vi "SUB-BLE Rx data (Debug)-CDC_KH2.vi"(8 "data in":u8[](array[numeric]) format="%2x") -> (2 "CDC debug":T1 caption="CDC Debugging data" {"Right Wing-C, C6/C0" format="%#.9f"; "Right Wing-B, C5/C0" format="%#.9f"; "Right Wing-A, C4/C0" format="%#.9f"; "Left Wing-C, C3/C0" format="%#.9f"; "Left Wing-B, C2/C0" format="%#.9f"; "Left Wing-A, C1/C0" format="%#.9f"}, 3 "CDC mon":T1 caption="CDC Monitoring data" {"Right Wing-C, C6/C0" format="%#.9f"; "Right Wing-B, C5/C0" format="%#.9f"; "Right Wing-A, C4/C0" format="%#.9f"; "Left Wing-C, C3/C0" format="%#.9f"; "Left Wing-B, C2/C0" format="%#.9f"; "Left Wing-A, C1/C0" format="%#.9f"})   [LabVIEW 2015]
doc: "Use this template to create an application that executes repeatedly until you click the Stop button. This template polls the state of the Stop button and does not use events. Use the Top-Level Application template (not available in the Base package) to create a single-loop application with event handling."
panel:
  out "BLE Packet (buf)":u8[](array[numeric])
  out "BLE Packet (data)":u8[](array[numeric])
  # "BLE 수신 데이터를 처리: Debugging data"
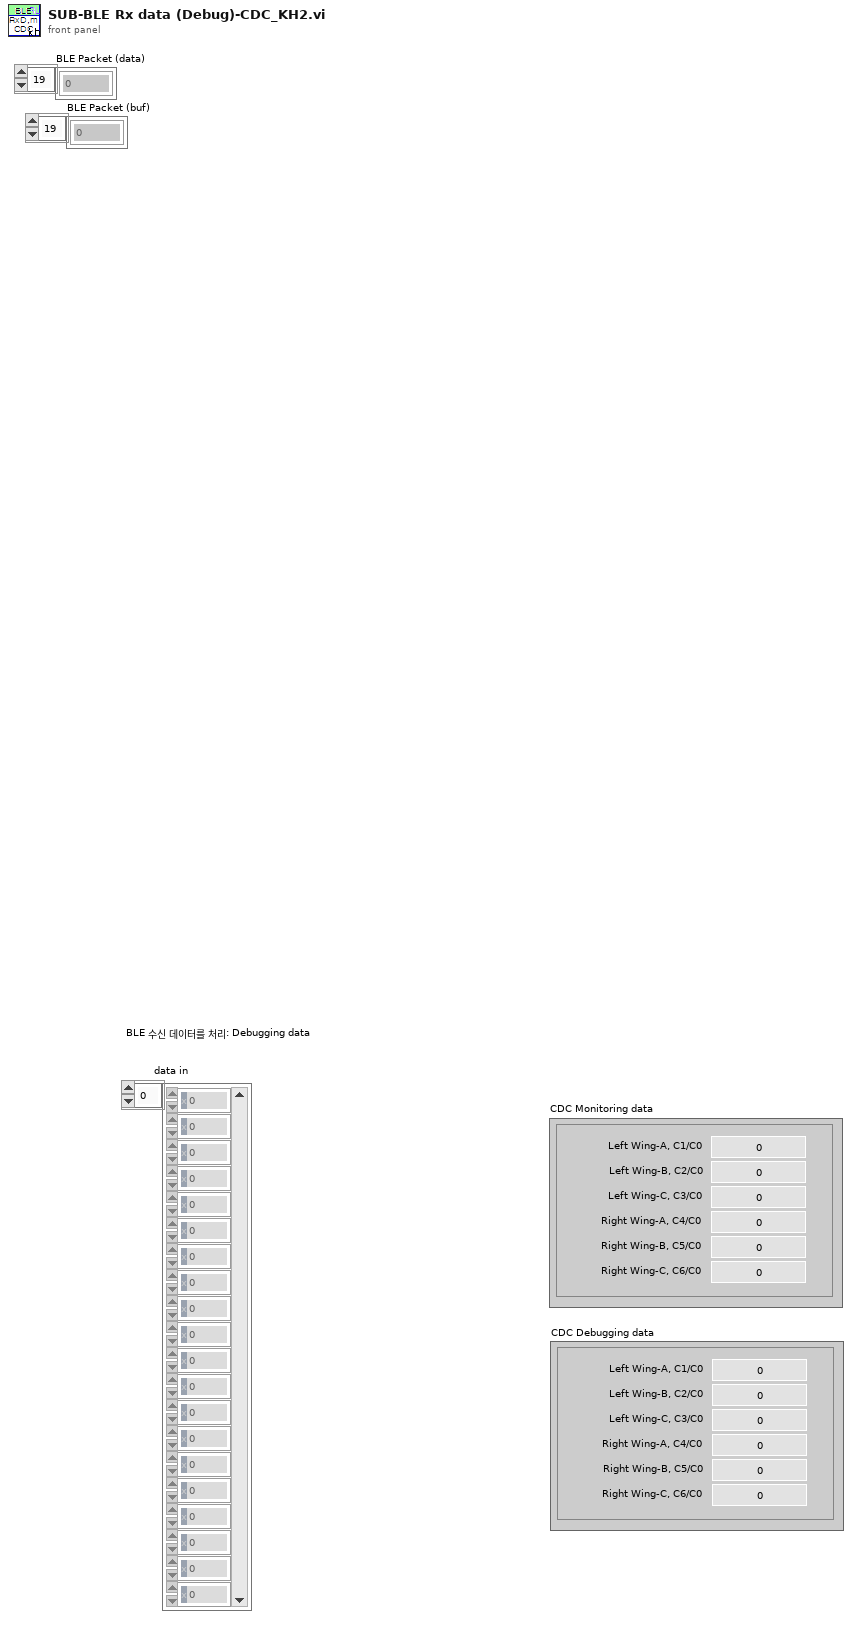
[diagram p1: front panel]
types:
  T1 = typedef "컨트롤-CDC data.ctl" = cluster{"Left Wing-A, C1/C0":dbl, "Left Wing-B, C2/C0":dbl, "Left Wing-C, C3/C0":dbl, "Right Wing-A, C4/C0":dbl, "Right Wing-B, C5/C0":dbl, "Right Wing-C, C6/C0":dbl}
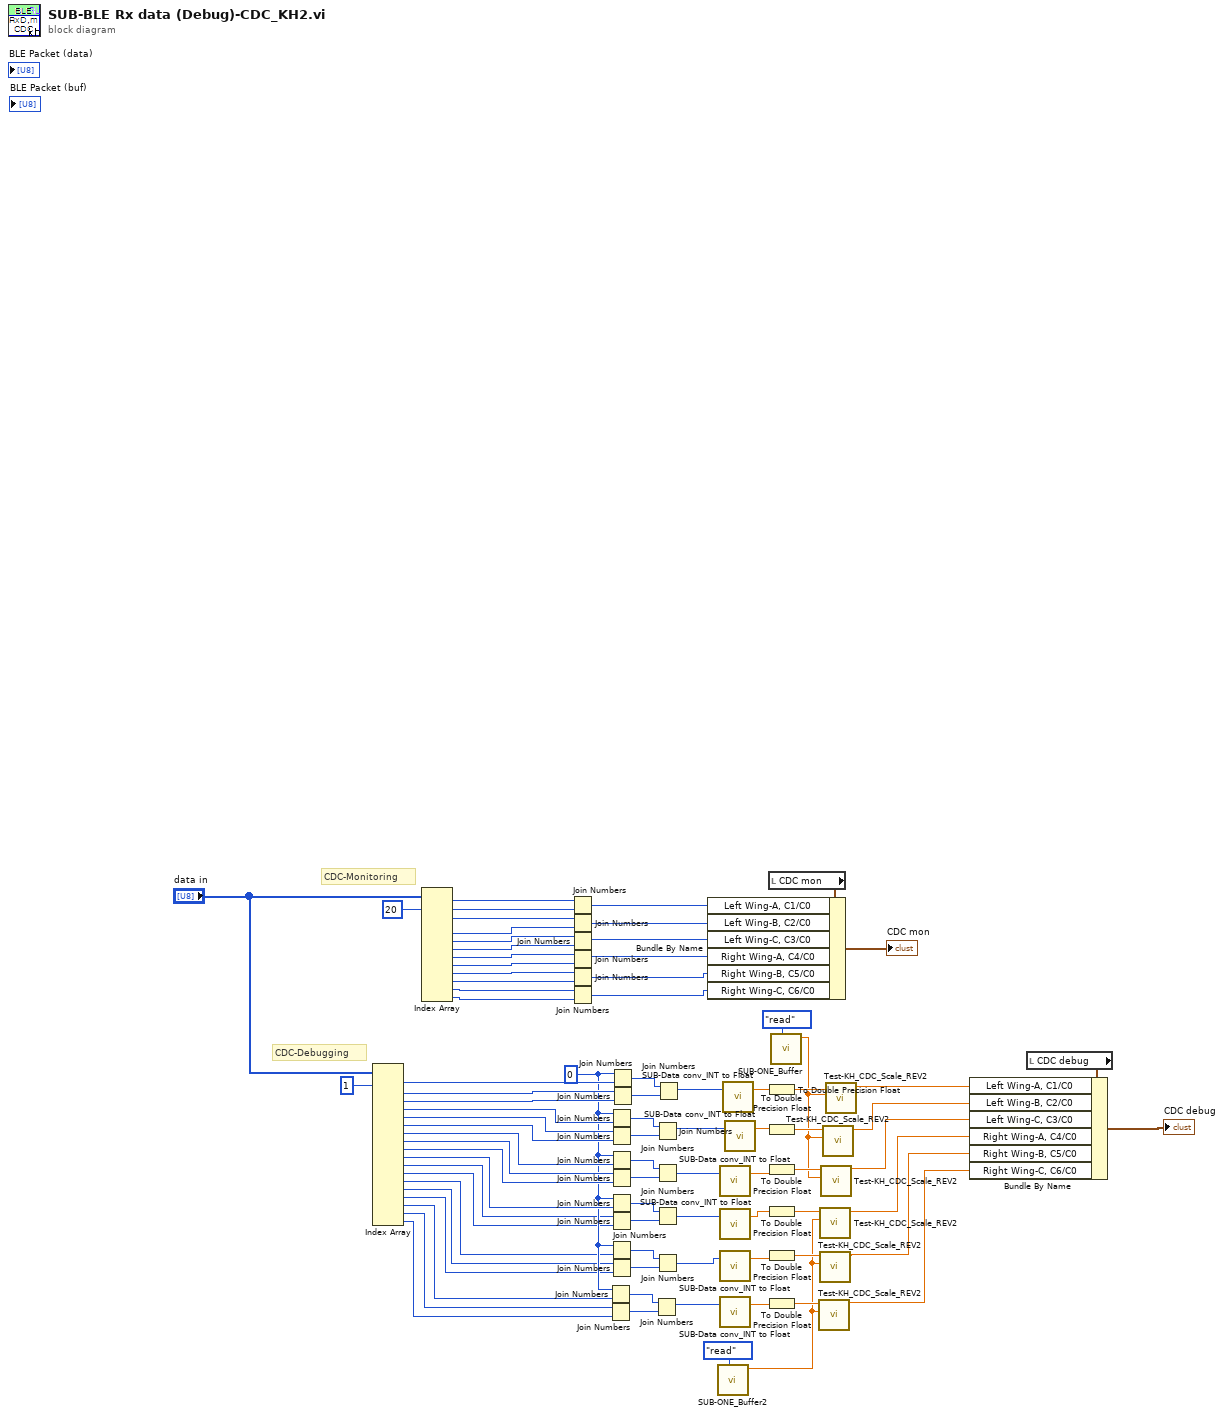
[diagram p0: block diagram]
diagram:
  w37 = u8 0 ("hi")
  # "CDC-Debugging"
  # "CDC-Monitoring"
  n1 = Index Array(array="data in", index #1=1 ("인덱스")) -> (element #1=w59:u8, element #2=w58:u8, element #3=w57:u8, element #4=w44:u8, element #5=w43:u8, element #6=w42:u8, element #7=w41:u8, element #8=w40:u8, element #9=w39:u8, element #10=w38:u8, element #11=w36:u8, element #12=w35:u8, element #13=w34:u8, element #14=w33:u8, element #15=w32:u8, element #16=w31:u8, element #17=w30:u8, element #18=w29:u8)  [unwired: 17 in]
  n2 = Index Array(array="data in", index #1=20 ("인덱스")) -> (element #1=w82:u8, element #2=w81:u8, element #3=w80:u8, element #4=w79:u8, element #5=w78:u8, element #6=w77:u8, element #7=w76:u8, element #8=w75:u8, element #9=w74:u8, element #10=w73:u8, element #11=w72:u8, element #12=w71:u8)  [unwired: 11 in]
  n3 = Join Numbers(hi=w82, lo=w81) -> ((hi.lo)=w69:u16)
  n4 = Join Numbers(hi=w80, lo=w79) -> ((hi.lo)=w68:u16)
  n5 = Join Numbers(hi=w78, lo=w77) -> ((hi.lo)=w67:u16)
  n6 = Join Numbers(hi=w76, lo=w75) -> ((hi.lo)=w66:u16)
  n7 = Join Numbers(hi=w74, lo=w73) -> ((hi.lo)=w65:u16)
  n8 = Join Numbers(hi=w72, lo=w71) -> ((hi.lo)=w64:u16)
  n9 = Join Numbers(hi=w37, lo=w31) -> ((hi.lo)=w46:u16)
  n10 = Join Numbers(hi=w30, lo=w29) -> ((hi.lo)=w45:u16)
  n11 = Join Numbers(hi=w37, lo=w44) -> ((hi.lo)=w54:u16)
  n12 = Join Numbers(hi=w43, lo=w42) -> ((hi.lo)=w53:u16)
  n13 = Join Numbers(hi=w37, lo=w41) -> ((hi.lo)=w51:u16)
  n14 = Join Numbers(hi=w40, lo=w39) -> ((hi.lo)=w52:u16)
  n15 = Join Numbers(hi=w37, lo=w38) -> ((hi.lo)=w50:u16)
  n16 = Join Numbers(hi=w36, lo=w35) -> ((hi.lo)=w49:u16)
  n17 = Join Numbers(hi=w37, lo=w34) -> ((hi.lo)=w47:u16)
  n18 = Join Numbers(hi=w33, lo=w32) -> ((hi.lo)=w48:u16)
  n19 = Join Numbers(hi=w37, lo=w59) -> ((hi.lo)=w55:u16)
  n20 = Join Numbers(hi=w58, lo=w57) -> ((hi.lo)=w56:u16)
  n21 = Join Numbers(hi=w46, lo=w45) -> ((hi.lo)=w27:u32)
  n22 = Join Numbers(hi=w54, lo=w53) -> ((hi.lo)=w24:u32)
  n23 = Join Numbers(hi=w51, lo=w52) -> ((hi.lo)=w25:u32)
  n24 = Join Numbers(hi=w50, lo=w49) -> ((hi.lo)=w26:u32)
  n25 = Join Numbers(hi=w47, lo=w48) -> ((hi.lo)=w28:u32)
  n26 = Join Numbers(hi=w55, lo=w56) -> ((hi.lo)=w23:u32)
  n27 = call "SUB-ONE_Buffer2.vi"("mode"=enum16{"write", "read"}."read") -> ("OUT"=w2:dbl)  [unwired: 10 in]
  n28 = call "SUB-Data conv_INT to Float.vi"("U32"=w25) -> ("FP32"=w18:sgl)  [unwired: 2 in]
  n29 = call "SUB-Data conv_INT to Float.vi"("U32"=w26) -> ("FP32"=w17:sgl)  [unwired: 2 in]
  n30 = call "SUB-Data conv_INT to Float.vi"("U32"=w28) -> ("FP32"=w16:sgl)  [unwired: 2 in]
  n31 = call "SUB-Data conv_INT to Float.vi"("U32"=w27) -> ("FP32"=w15:sgl)  [unwired: 2 in]
  n32 = call "SUB-Data conv_INT to Float.vi"("U32"=w23) -> ("FP32"=w22:sgl)  [unwired: 2 in]
  n33 = call "SUB-Data conv_INT to Float.vi"("U32"=w24) -> ("FP32"=w19:sgl)  [unwired: 2 in]
  n34 = To Double Precision Float(number=w22) -> (double precision float=w20:dbl)
  n35 = To Double Precision Float(number=w19) -> (double precision float=w14:dbl)
  n36 = To Double Precision Float(number=w18) -> (double precision float=w13:dbl)
  n37 = To Double Precision Float(number=w17) -> (double precision float=w12:dbl)
  n38 = To Double Precision Float(number=w16) -> (double precision float=w11:dbl)
  n39 = To Double Precision Float(number=w15) -> (double precision float=w10:dbl)
  n40 = local read "CDC mon"() -> (w84:T1)
  n41 = Bundle By Name(cluster=w84, "Left Wing-A, C1/C0"=w69, "Left Wing-B, C2/C0"=w68, "Left Wing-C, C3/C0"=w67, "Right Wing-A, C4/C0"=w66, "Right Wing-B, C5/C0"=w65, "Right Wing-C, C6/C0"=w64) -> (→"CDC mon":T1)
  n42 = call "SUB-ONE_Buffer.vi"("mode"=enum16{"write", "read"}."read") -> ("OUT"=w1:dbl)  [unwired: 10 in]
  n43 = call "Test-KH_CDC_Scale_REV2.vi"("Scale"=w2, "r"=w10) -> ("2byte"=w5:dbl)  [unwired: 9 in]
  n44 = call "Test-KH_CDC_Scale_REV2.vi"("Scale"=w2, "r"=w12) -> ("2byte"=w7:dbl)  [unwired: 9 in]
  n45 = call "Test-KH_CDC_Scale_REV2.vi"("Scale"=w2, "r"=w11) -> ("2byte"=w6:dbl)  [unwired: 9 in]
  n46 = call "Test-KH_CDC_Scale_REV2.vi"("Scale"=w1, "r"=w13) -> ("2byte"=w8:dbl)  [unwired: 9 in]
  n47 = call "Test-KH_CDC_Scale_REV2.vi"("Scale"=w1, "r"=w14) -> ("2byte"=w9:dbl)  [unwired: 9 in]
  n48 = call "Test-KH_CDC_Scale_REV2.vi"("Scale"=w1, "r"=w20) -> ("2byte"=w21:dbl)  [unwired: 9 in]
  n49 = local read "CDC debug"() -> (w62:T1)
  n50 = Bundle By Name(cluster=w62, "Left Wing-A, C1/C0"=w21, "Left Wing-B, C2/C0"=w9, "Left Wing-C, C3/C0"=w8, "Right Wing-A, C4/C0"=w7, "Right Wing-B, C5/C0"=w6, "Right Wing-C, C6/C0"=w5) -> (→"CDC debug":T1)
